vi "Text0006.vi"   [LabVIEW 2013]
uses:
  <vilib>/Heliosphere Research LLC/Advanced Plotting Toolkit/api_core/NewPlotScales.ctl
  <vilib>/Heliosphere Research LLC/Advanced Plotting Toolkit/Advanced Plotting Toolkit.lvlib
types:
  T1 = typedef "Advanced Plotting Toolkit.lvlib/NewPlotScales.ctl" = enum16{"Default", "Linear", "Log", "Symlog"}
  T2 = typedef "Advanced Plotting Toolkit.lvlib/PlotID.ctl" = i32
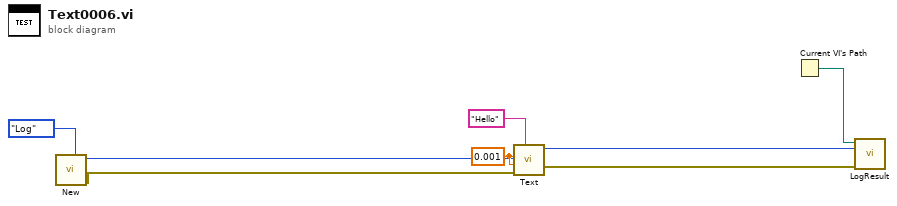
[diagram p0: block diagram]
diagram:
  w7 = 0.001 ("X Position")
  n1 = call <vilib>:"New.vi"("Y Axis Scale"=NewPlotScales."Log") -> ("error out"=w2:errorcluster, "Plot ID"=w3:T2)  [unwired: 9 in]
  n2 = call <vilib>:"Text.vi"("Text"="Hello", "error in (no error)"=w2, "Y Position"=w7, "X Position"=w7, "Plot ID"=w3) -> ("error out"=w4:errorcluster, "Plot ID Out"=w5:T2)  [unwired: 5 in]
  n3 = Current VI's Path() -> (path=w8:path)
  n4 = call "LogResult.vi"("Test Result"=w4, "Test Artifact"=w5, "VI Path"=w8) -> ()  [unwired: 9 in]
